vi "Place Orders.vi"(8 "error in (no error)":errorcluster, 10 "Items":refnum<class "Order Item.lvclass">[](array[class]), 11 "Cashier in":refnum<class "Cashier.lvclass">) -> (0 "error out":errorcluster, 3 "Cashier out":refnum<class "Cashier.lvclass">)   [LabVIEW 2020, in "Cashier.lvclass"]
uses:
  Cashier.lvclass
  Support/Order Item/Order Item.lvclass
  C:/git/astemes-triarc-examples/source/Coffee Shop/Processes/People/Workers/Worker/Worker.lvclass
  C:/git/astemes-triarc-examples/source/Coffee Shop/Processes/People/Person/Person.lvclass
  Worker/Worker.lvclass/Worker.ctl
  Person/Person.lvclass/Person.ctl
  Process Job/Job Handler.lvclass
  Worker/Worker.lvclass
  Person/Person.lvclass
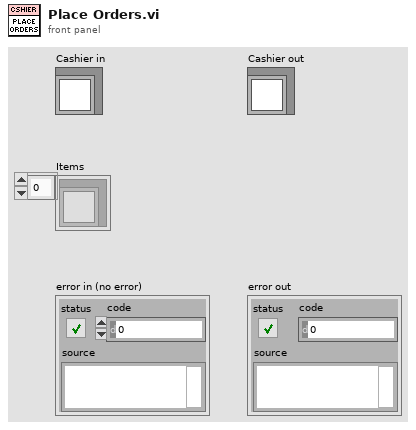
[diagram p1: front panel]
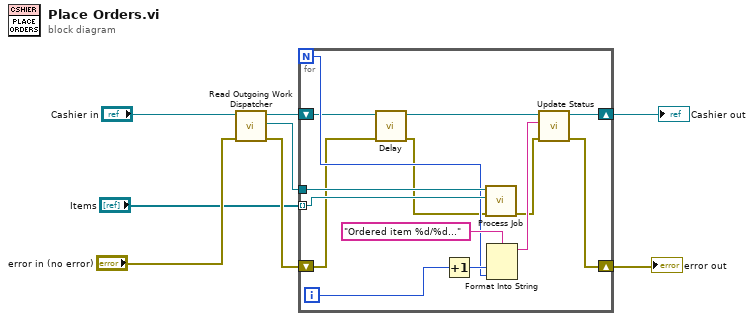
[diagram p0: block diagram]
diagram:
  n1 = call "Read Outgoing Work Dispatcher.vi"("error in (no error)"="error in (no error)", "Worker In"="Cashier in") -> ("error out"=w8:errorcluster, "Job Handler"=w4:refnum<class "Job Handler.lvclass">, "Worker Out"=w2:refnum<class "Cashier.lvclass">)  [unwired: 7 in]
  n2 = for {
    N -> [w17]
    tunnel: w4 -> [w22]
    tunnel: "Items" -> [w21] mode=indexing
    shift-right: [w16] -> w6
    shift-left: w8 -> [w11]
    shift-right: [w15] -> w1
    shift-left: w2 -> [w13]
    i -> [w19]
    n3 = call "Delay.vi"("error in (no error)"=w11, "Person In"=w13) -> ("error out"=w10:errorcluster, "Person Out"=w12:refnum<class "Cashier.lvclass">)  [unwired: 8 in]
    n4 = Increment(x=w19) -> (x+1=w20:i32)
    n5 = call-dynamic "Process Job.vi"("error in (no error)"=w10, "Job"=w21, "Process Job In"=w22) -> ("error out"=w9:errorcluster)  [unwired: 7 in, 1 out]
    n6 = Format Into String(format string="Ordered item %d/%d..." ("Ordered Item"), w20, w17) -> (resulting string=w14:string)  [unwired: 2 in, 1 out]
    n7 = call "Update Status.vi"("error in (no error)"=w9, "Status"=w14, "Person In"=w12) -> ("error out"=w16:errorcluster, "Person Out"=w15:refnum<class "Cashier.lvclass">)  [unwired: 7 in]
  }
  "error out" <- w6
  "Cashier out" <- w1
